vi "Getter.vi"(8 "Error In":errorcluster, 11 "Waypoint In":refnum<class "Waypoint.lvclass">) -> (0 "Error Out":errorcluster, 1 "Coords":T1 {"North" format="%#_10f"; "East" format="%#_8f"}, 2 "Tolerance (meters?)":dbl, 3 "Waypoint Out":refnum<class "Waypoint.lvclass">, 4 "Sailing Point?":bool, 5 "Done?":bool)   [LabVIEW 2013, in "Waypoint.lvclass"]
doc: "A getter vi for waypoint class\n\nMac-I Crowell\nJanuray 2014"
uses:
  Waypoint.lvclass
  Data/TypeDefs/UTM Location.ctl
  Waypoint.lvclass/Waypoint.ctl
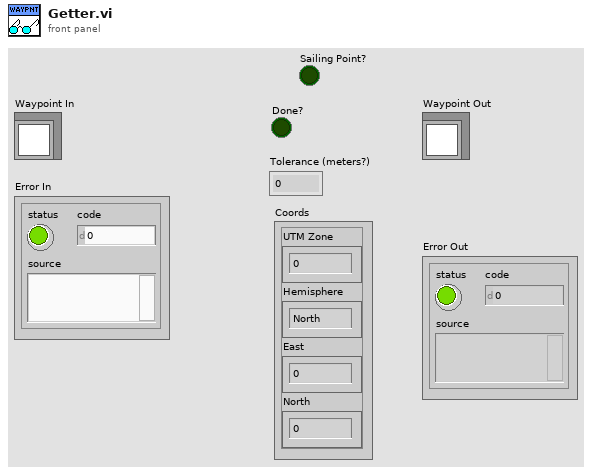
[diagram p1: front panel]
types:
  T1 = typedef "UTM Location.ctl" = cluster{"UTM Zone":dbl, "Hemisphere":enum16{"North", "South"}, "East":dbl, "North":dbl}
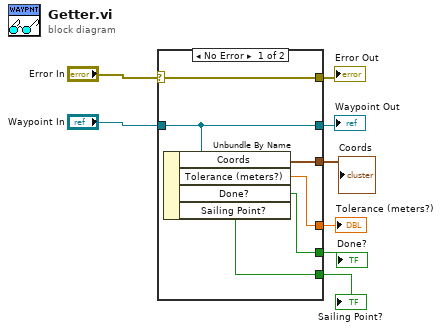
[diagram p0: block diagram]
diagram:
  n1 = case shown="No Error" "Error In" {
    selector: "Error In" -> [w14 w15]
    tunnel: [w14 w15] -> w6
    tunnel: "Waypoint In" -> [w13 w16]
    tunnel: [w13 w16] -> w8
    tunnel: [w12 _] -> w2
    tunnel: [w11 _] -> w4
    tunnel: [w10 _] -> w3
    tunnel: [w9 _] -> w1
    frame No Error {
      n2 = Unbundle By Name(w13) -> ("Coords"=w12:T1, "Tolerance (meters?)"=w10:dbl, "Done?"=w11:bool, "Sailing Point?"=w9:bool)
    }
    frame Error {
    }
  }
  "Waypoint Out" <- w8
  "Error Out" <- w6
  "Done?" <- w4
  "Tolerance (meters?)" <- w3
  "Coords" <- w2
  "Sailing Point?" <- w1
